vi "Words To Network-Order Bytes I64.vi"(1 "word":i64 format="%016x") -> (0 "bytes":u8[](array[numeric]) format="%02x")   [LabVIEW 2020, in "NI_Bit Manipulation.lvlib"]
uses:
  <vilib>/Bit Manipulation/NI_Bit Manipulation.lvlib
  3451642c-1dfe-4f1f-97de-8771b4fa65f6.vi
  3451642c-1dfe-4f1f-97de-8771b4fa65f6.vi/cae554d2-4c7f-3fea-a807-6b7b33d6ca3f.vi
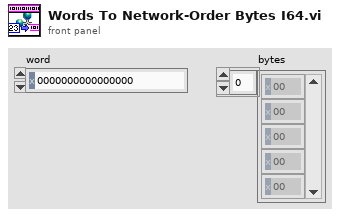
[diagram p1: front panel]
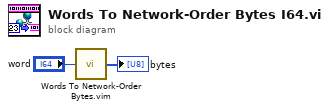
[diagram p0: block diagram]
diagram:
  n1 = call "Words To Network-Order Bytes.vim"("word"="word") -> ("bytes"=→"bytes":u8[])
